vi "影像辨識.vi"() -> ()   [LabVIEW 2014]
uses:
  <vilib>/vision/NI_Vision_Development_Module.lvlib
panel:
  out "後":u32[][](array[numeric])
  out "Image Pixels (U32) 2":u32[][](array[numeric])
  out "Image 2":T1(plugin-control)
  out "Array":u32[][](array[colorbox])
  out "«e":u32[][](array[numeric]) format="%x"
  out "Image":T1(plugin-control)
  in  "Stop (F)":bool
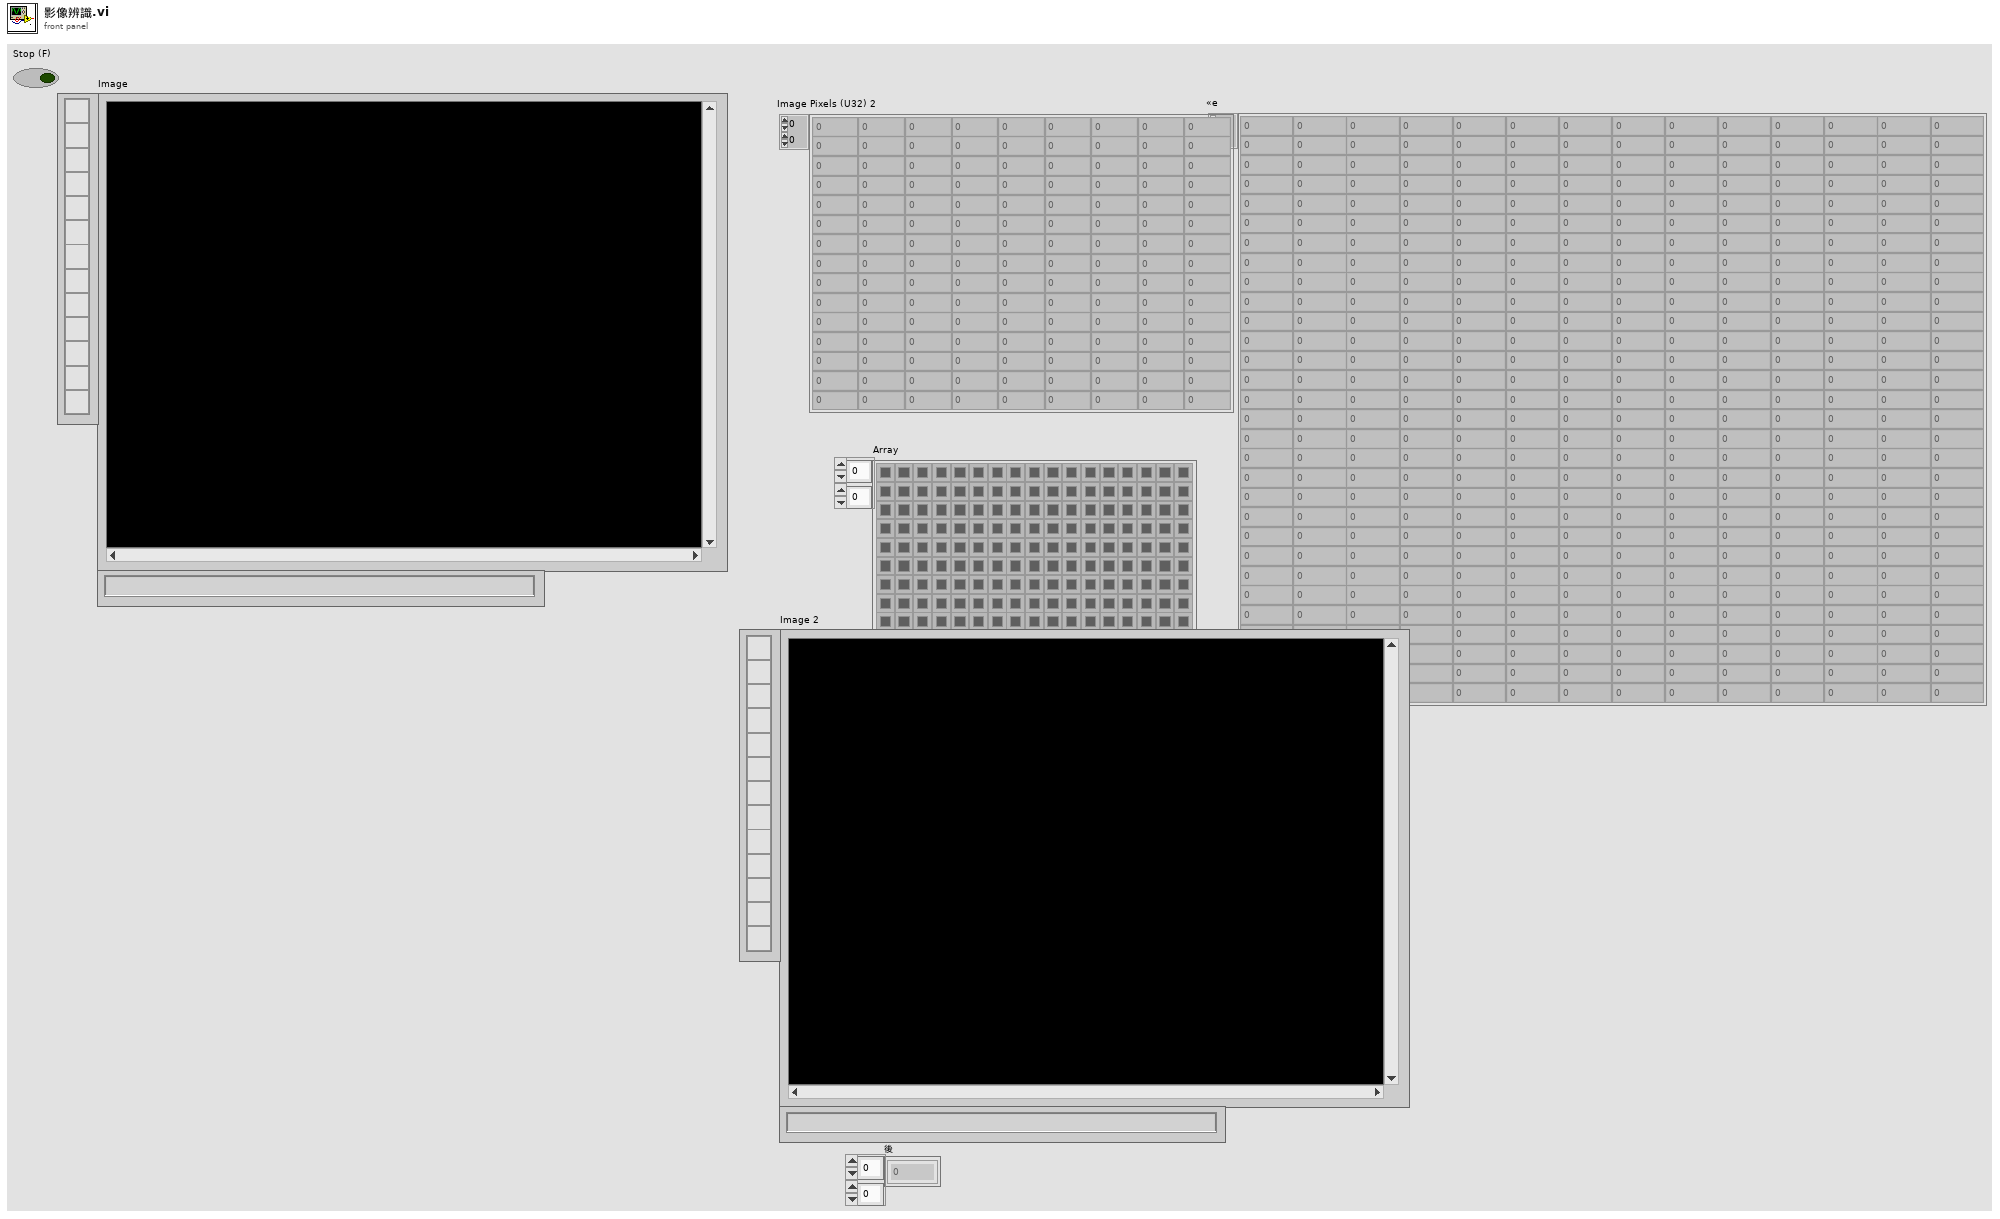
[diagram p1: front panel]
types:
  T1 = typedef "IMAQ Image.ctl" = refnum<image>
  T2 = typedef "Image Type" = u32
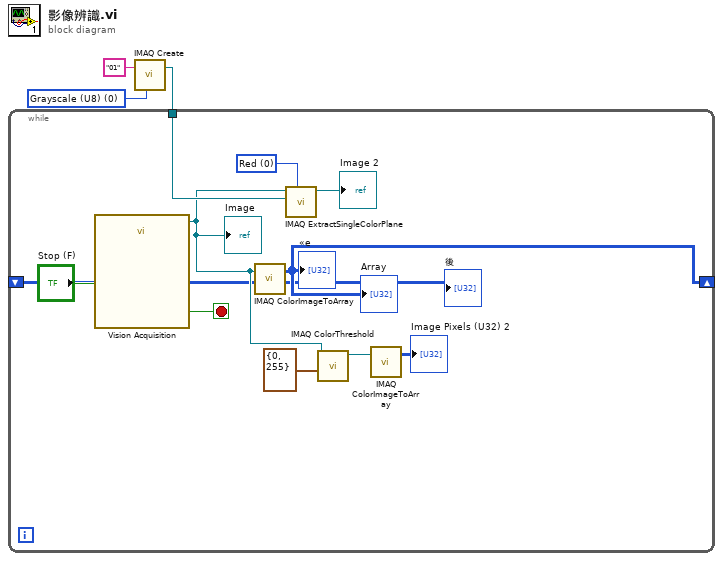
[diagram p0: block diagram]
diagram:
  w2 = T2 0 items=["Grayscale (U8)", "Grayscale (I16)", "Grayscale (SGL)", "Complex (CSG)", "RGB (U32)", "HSL (U32)", "RGB (U64)", "Grayscale (U16)"] ("Image Type")
  n1 = call "IMAQ Create"("Image Name"="01", "Image Type"=w2) -> ("New Image"=w3:T1)  [unwired: 3 in, 1 out]
  n2 = while {
    tunnel: w3 -> [w12]
    shift-right: [w5] -> _
    shift-left: _ -> [w4]
    stop <- w13 stop-if-true
    w11 = 0 items=["Red", "Green", "Blue", "Hue", "Saturation", "Luminance", "Value", "Intensity"] ("Color Plane")
    n3 = call "Vision Acquisition"("Stop (F)"="Stop (F)") -> ("Image Out"=w6:T1, "Stopped"=w13:bool)  [unwired: 24 in, 1 out]
    "Image" <- w6
    n4 = call "IMAQ ColorImageToArray"("Image"=w6) -> ("Image Pixels (U32)"=w5:u32[][])  [unwired: 3 in, 2 out]
    "«e" <- w5
    "Array" <- w5
    n5 = call "IMAQ ExtractSingleColorPlane"("Color Plane"=w11, "Image Dst"=w12, "Image Src"=w6) -> ("Image Dst Out"=→"Image 2":T1)  [unwired: 7 in, 1 out]
    n6 = call "IMAQ ColorThreshold"("Red or Hue Range"=cluster{"Lower value":i32, "Upper value":i32} {"Lower value"=0, "Upper value"=255}, "Image Src"=w6) -> ("Image Dst Out"=w8:T1)  [unwired: 8 in, 1 out]
    n7 = call "IMAQ ColorImageToArray"("Image"=w8) -> ("Image Pixels (U32)"=→"Image Pixels (U32) 2":u32[][])  [unwired: 3 in, 2 out]
    "後" <- w4
  }
